vi "Test DataPoint Generation.vi"() -> ()   [LabVIEW 2018, in "InfluxDB Client.lvlib"]
uses:
  Controls/FieldSet.ctl
  Controls/TagSet.ctl
  Classes/DataPoint/DataPoint.lvclass/DataPoint.ctl
  InfluxDB Client.lvlib
  Classes/DataPoint/DataPoint.lvclass
panel:
  out "Line Protocol":string
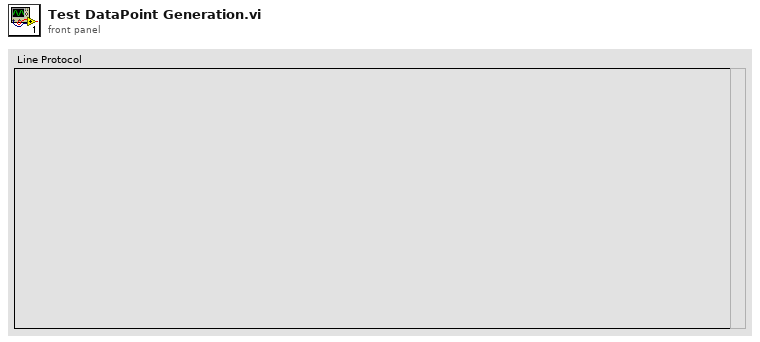
[diagram p1: front panel]
types:
  T1 = typedef "InfluxDB Client.lvlib/TagSet.ctl" = cluster{"Key":string, "Value":string}
  T2 = typedef "InfluxDB Client.lvlib/FieldSet.ctl" = cluster{"Key":string, "Value":variant}
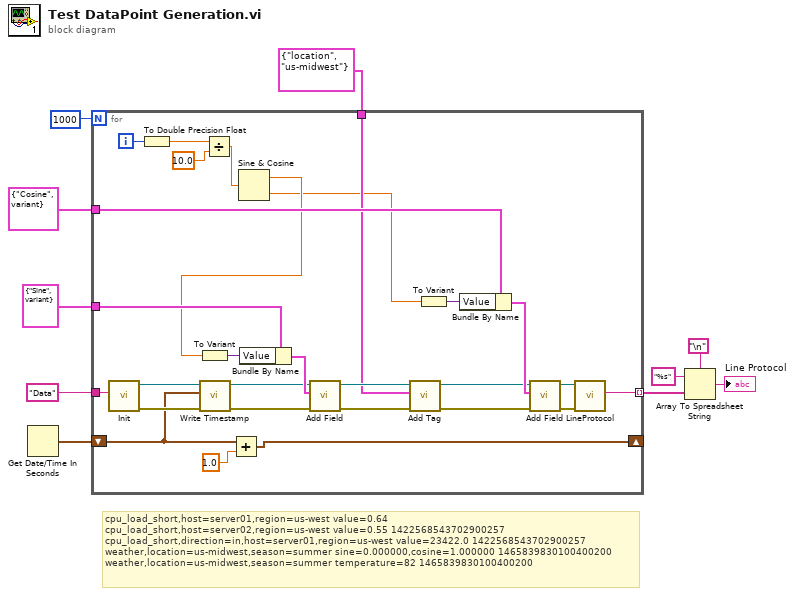
[diagram p0: block diagram]
diagram:
  # "cpu_load_short,host=server01,region=us-west value=0.64 \ncpu_load_short,host=server02,region=us-west value=0.55 1422568543702900257\ncpu_load_short,direction=in,host=server01,region=us-west value=23422.0 1422568543702900257\nweather,location=us-midwest,season=summer sine=0.000000,cosine=1.000000 1465839830100400200\nweather,location=us-midwest,season=summer temperature=82 1465839830100400200"
  n1 = Get Date/Time In Seconds() -> (seconds since 1Jan1904=w5:timestamp)
  n2 = for {
    N: 1000 -> [_]
    tunnel: T2 {"Key"="Sine", "Value"=variant} ("FieldSet") -> [w31]
    tunnel: T2 {"Key"="Cosine", "Value"=variant} ("FieldSet") -> [w30]
    tunnel: T1 {"Key"="location", "Value"="us-midwest"} ("TagSet") -> [w27]
    tunnel: "Data" ("Measurement") -> [w24]
    tunnel: [w18] -> w4 mode=indexing
    shift-right: [w11] -> _
    shift-left: w5 -> [w13]
    i -> [w38]
    n3 = call "Init.vi"("Measurement"=w24) -> ("error out"=w15:errorcluster, "DataPoint out"=w16:refnum<class "DataPoint.lvclass">)  [unwired: 9 in]
    n4 = To Double Precision Float(number=w38) -> (double precision float=w37:dbl)
    n5 = call "Write Timestamp.vi"("error in (no error)"=w15, "Timestamp"=w13, "DataPoint in"=w16) -> ("error out"=w14:errorcluster, "DataPoint out"=w17:refnum<class "DataPoint.lvclass">)  [unwired: 7 in]
    n6 = Divide(x=w37, y=10.0) -> (x/y=w23:dbl)
    n7 = Add(x=w13, y=1.0) -> (x+y=w11:timestamp)
    n8 = Sine & Cosine(0:w23) -> (1:w22:dbl, 2:w21:dbl)
    n9 = To Variant(anything=w22) -> (Variant=w32:variant)
    n10 = Bundle By Name(cluster=w31, "Value"=w32) -> (w33:T2)
    n11 = call "Add Field.vi"("error in (no error)"=w14, "FieldSet"=w33, "DataPoint in"=w17) -> ("error out"=w28:errorcluster, "DataPoint out"=w29:refnum<class "DataPoint.lvclass">)  [unwired: 7 in]
    n12 = call "Add Tag.vi"("error in (no error)"=w28, "TagSet"=w27, "DataPoint in"=w29) -> ("error out"=w25:errorcluster, "DataPoint out"=w26:refnum<class "DataPoint.lvclass">)  [unwired: 7 in]
    n13 = To Variant(anything=w21) -> (Variant=w34:variant)
    n14 = Bundle By Name(cluster=w30, "Value"=w34) -> (w35:T2)
    n15 = call "Add Field.vi"("error in (no error)"=w25, "FieldSet"=w35, "DataPoint in"=w26) -> ("error out"=w19:errorcluster, "DataPoint out"=w20:refnum<class "DataPoint.lvclass">)  [unwired: 7 in]
    n16 = call "LineProtocol.vi"("error in (no error)"=w19, "DataPoint in"=w20) -> ("Line protocol"=w18:string)  [unwired: 7 in, 2 out]
  }
  n17 = Array To Spreadsheet String(delimiter (Tab)="\n", array=w4, 3:"%s" ("format string")) -> (spreadsheet string=→"Line Protocol":string)
